vi "Client Begin Bidirectional Streaming Call.vi"(5 "Response Message Name":string, 7 "Request Message Name":string, 8 "error in":errorcluster, 9 "timeout (ms)":i32=-1, 10 "Method Name":string, 11 "ClientID in":T1) -> (0 "error out":errorcluster, 2 "Call ID out":T1, 3 "ClientID out":T1)   [LabVIEW 2019, in "grpc-lvsupport.lvlib"]
uses:
  grpc-lvsupport.lvlib
  Shared/grpcId.ctl
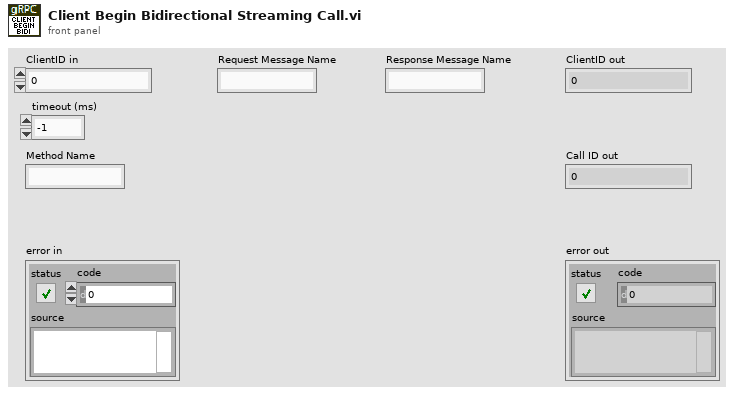
[diagram p1: front panel]
types:
  T1 = typedef "grpc-lvsupport.lvlib/grpcId.ctl" = u64
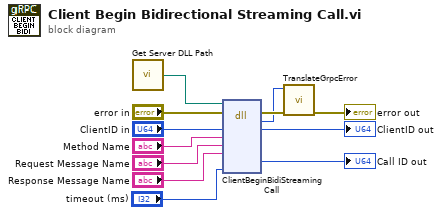
[diagram p0: block diagram]
diagram:
  n1 = call "Get Server DLL Path.vi"() -> ("Server dll path"=w11:path)
  n2 = dll-call lib="?" fn="ClientBeginBidiStreamingCall"(path in=w11, error in="error in", "ClientId"="ClientID in", "methodName"="Method Name", "requestMessageName"="Request Message Name", "responseMessageName"="Response Message Name", "timeoutMs"="timeout (ms)") -> (error out=w4:errorcluster, "return type"=w2:i32, "ClientId"=→"ClientID out":u64, "callId"=→"Call ID out":u64)  [unwired: 6 in, 1 out]
  n3 = call "TranslateGrpcError.vi"("error in"=w4, "Error Code"=w2) -> ("error out"=→"error out":errorcluster)  [unwired: 9 in]
